vi "V2int16.vi"(4 "InV":dbl) -> (1 "Out i16":i16)   [LabVIEW 2013]
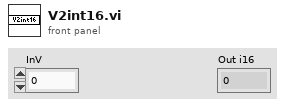
[diagram p1: front panel]
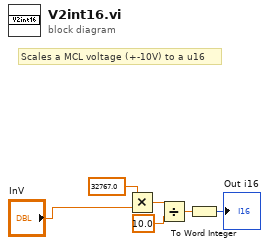
[diagram p0: block diagram]
diagram:
  # "Scales a MCL voltage (+-10V) to a u16"
  n1 = Multiply(x=32767.0 ("y"), y="InV") -> (x*y=w4:dbl)
  n2 = Divide(x=w4, y=10.0) -> (x/y=w2:dbl)
  n3 = To Word Integer(number=w2) -> (16bit integer=→"Out i16":i16)
